vi "[RT]CTRL_Heater.vi"(11 "target-temp":dbl) -> (3 "temp_reached":bool)   [LabVIEW 2018]
uses:
  [GlobVar]SensorState.vi
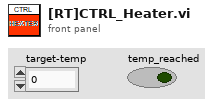
[diagram p1: front panel]
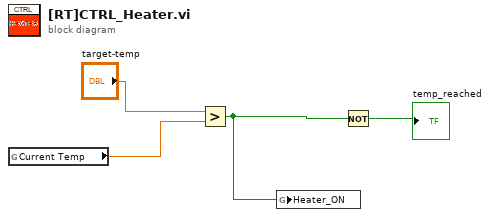
[diagram p0: block diagram]
diagram:
  n1 = global read "[GlobVar]SensorState.vi" "Current Temp"() -> (w4:dbl)
  n2 = Greater?(x="target-temp", y=w4) -> (0:w1:bool)
  n3 = global write "[GlobVar]SensorState.vi" "Heater_ON"(w1) -> ()
  n4 = Not(x=w1) -> (.not. x?=→"temp_reached":bool)
